vi "build.key.maps.vi"() -> ()   [LabVIEW 2024]
uses:
  definitions/comicvine_issue.generic_credit.ctl
  definitions/local_issue.ctl
  definitions/comicvine_issue.associated_image.ctl
  definitions/comicvine_issue.person_credit.ctl
  <vilib>/addons/_JKI.lib/Serialization/JSON/JKI JSON Serialization.lvlib
panel:
  out "progress":i32(slide) scale=0.0..21267.0
  out "current file":string
  in  "error in (no error)":errorcluster
  out "error out":errorcluster
  in  "storyArc map path":path=path "D:/Comics/data/key_maps/storyArc.json"
  in  "team map path":path=path "D:/Comics/data/key_maps/team.json"
  in  "character map path":path=path "D:/Comics/data/key_maps/char.json"
  in  "Folder Path":path=path "D:/Comics/data/cv_issues"
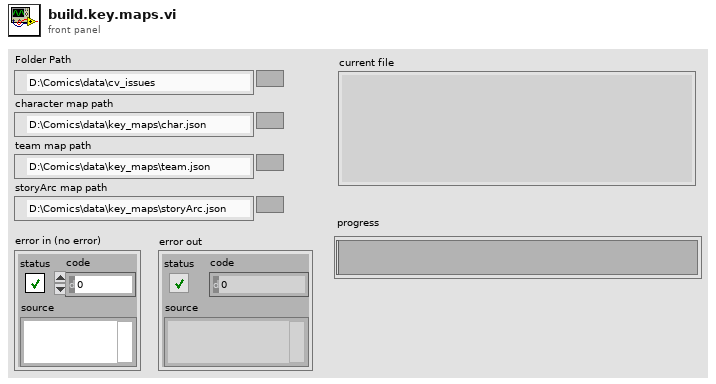
[diagram p1: front panel]
types:
  T1 = typedef "comicvine_issue.generic_credit.ctl" = cluster{"id":i32, "name":string}
  T2 = cluster{"map":cluster{"key":T1, "issue_ids":i32[]}[]}
  T3 = typedef "local_issue.ctl" = cluster{"cover_date":timestamp, "id":i32, "cv_id":string, "name":string, "sortable_name":string, "issue_number":string, "deck":string, "description":string, "volume":T1, "store_date":timestamp, "date_last_updated":timestamp, "site_detail_url":string, "cover_url":string, "associated_images":T4[], "characters":T1[], "concepts":T1[], "creators":T5[], "storyArcs":T1[], "teams":T1[]}
  T4 = typedef "comicvine_issue.associated_image.ctl" = cluster{"original_url":string, "id":i32}
  T5 = typedef "comicvine_issue.person_credit.ctl" = cluster{"id":i32, "name":string, "role":string}
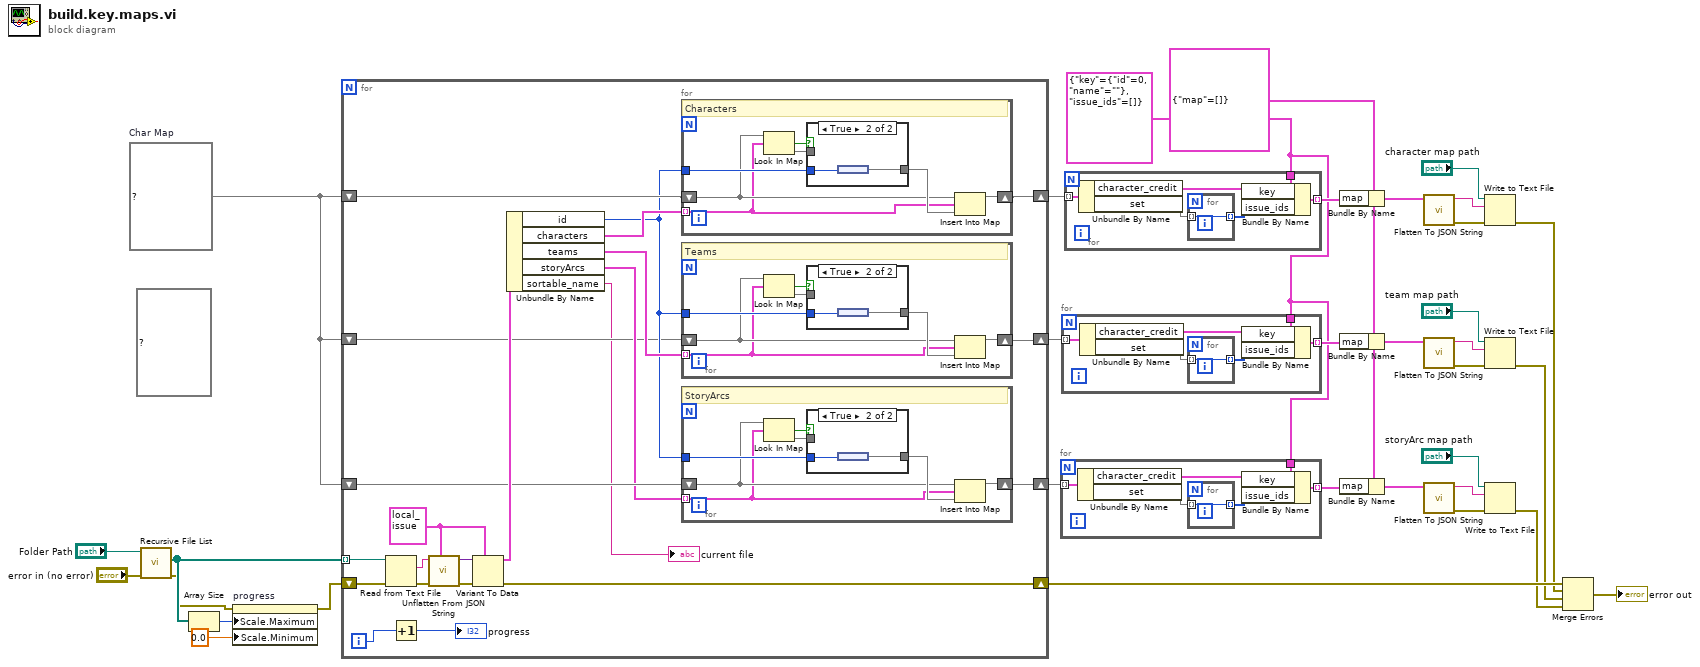
[diagram p0: block diagram]
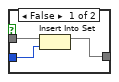
[diagram p2: hidden frame]
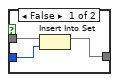
[diagram p3: hidden frame]
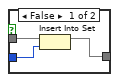
[diagram p4: hidden frame]
diagram:
  w6 = T2 {"map"=[]}
  w7 = cluster{"key":T1, "issue_ids":i32[]} {"key"={"id"=0, "name"=""}, "issue_ids"=[]}
  w8 = map{T1, set{i32}} {}  # Char Map
  (unwired) map{i32, set{i32}} {} ("map")
  n1 = call <vilib>:"Recursive File List.vi"("error in (no error)"="error in (no error)", "Folder Path"="Folder Path") -> ("error out"=w2:errorcluster, "All Files in Dir"=w5:path[])  [unwired: 5 in, 3 out]
  n2 = Array Size(array=w5) -> (size(s)=w4:i32)
  n3 = property on="progress" class="Slide (strict)"(error in=w2, "Scale.Maximum"=w4, "Scale.Minimum"=0.0 ("Scale.Range:Minimum")) -> (error out=w1:errorcluster)  [unwired: 1 in, 1 out]
  n4 = for {
    shift-right: [w48] -> w14
    shift-left: w1 -> [w54]
    tunnel: w5 -> [w55] mode=indexing
    shift-right: [w45] -> w32
    shift-left: w8 -> [w46]
    shift-right: [w39] -> w16
    shift-left: w8 -> [w37]
    shift-right: [w38] -> w15
    shift-left: w8 -> [w43]
    i -> [w35]
    w50 = T3 {"cover_date"=timestamp(0 s since 1904-01-01), "id"=0, "cv_id"="", "name"="", "sortable_name"="", "issue_number"="", "deck"="", "description"="", "volume"={"id"=0, "name"=""}, "store_date"=timestamp(0 s since 1904-01-01), "date_last_updated"=timestamp(0 s since 1904-01-01), "site_detail_url"="", "cover_url"="", "associated_images"=[], "characters"=[], "concepts"=[], "creators"=[], "storyArcs"=[], "teams"=[]} ("issue")
    n5 = Read from Text File(file (use dialog)=w55, error in=w54) -> (text=w52:string, error out=w53:errorcluster)  [unwired: 2 in, 2 out]
    n6 = Increment(x=w35) -> (x+1=→"progress":i32)
    n7 = call <vilib>:"Unflatten From JSON String.vi"("Type and Defaults"=w50, "error in"=w53, "JSON String"=w52) -> ("error out"=w49:errorcluster, "Variant"=w51:variant)  [unwired: 7 in]
    n8 = Variant To Data(error in=w49, type=w50, Variant=w51) -> (data=w47:T3, error out=w48:errorcluster)
    n9 = Unbundle By Name(w47) -> ("id"=w40:i32, "characters"=w44:T1[], "teams"=w41:T1[], "storyArcs"=w42:T1[], "sortable_name"=→"current file":string)
    n10 = for {
      tunnel: w44 -> [w80] mode=indexing
      shift-right: [w82] -> w45
      shift-left: w46 -> [w81]
      tunnel: w40 -> [w84]
      # "Characters"
      n11 = Look In Map(map=w81, key=w80) -> (key not found?=w86:bool, value=w85:set{i32})  [unwired: 1 in]
      n12 = case shown="True" w86 {
        tunnel: w85 -> [w89 _]
        tunnel: w84 -> [w88 w91]
        tunnel: [w87 w90] -> w83
        frame False {
          n13 = Insert Into Set(10:w88, 11:w89) -> (3:w87:set{i32})  [unwired: 1 out]
        }
        frame True {
          n14 = node(w91) -> (w90:set{i32})
        }
      }
      n15 = Insert Into Map(map in=w81, key=w80, value=w83) -> (map out=w82:map{T1, set{i32}})  [unwired: 2 out]
    }
    n16 = for {
      tunnel: w41 -> [w68] mode=indexing
      shift-right: [w70] -> w39
      shift-left: w37 -> [w69]
      tunnel: w40 -> [w72]
      # "Teams"
      n17 = Look In Map(map=w69, key=w68) -> (key not found?=w74:bool, value=w73:set{i32})  [unwired: 1 in]
      n18 = case shown="True" w74 {
        tunnel: w73 -> [w77 _]
        tunnel: w72 -> [w76 w79]
        tunnel: [w75 w78] -> w71
        frame False {
          n19 = Insert Into Set(10:w76, 11:w77) -> (3:w75:set{i32})  [unwired: 1 out]
        }
        frame True {
          n20 = node(w79) -> (w78:set{i32})
        }
      }
      n21 = Insert Into Map(map in=w69, key=w68, value=w71) -> (map out=w70:map{T1, set{i32}})  [unwired: 2 out]
    }
    n22 = for {
      tunnel: w42 -> [w56] mode=indexing
      shift-right: [w58] -> w38
      shift-left: w43 -> [w57]
      tunnel: w40 -> [w60]
      # "StoryArcs"
      n23 = Look In Map(map=w57, key=w56) -> (key not found?=w62:bool, value=w61:set{i32})  [unwired: 1 in]
      n24 = case shown="True" w62 {
        tunnel: w61 -> [w65 _]
        tunnel: w60 -> [w64 w67]
        tunnel: [w63 w66] -> w59
        frame False {
          n25 = Insert Into Set(10:w64, 11:w65) -> (3:w63:set{i32})  [unwired: 1 out]
        }
        frame True {
          n26 = node(w67) -> (w66:set{i32})
        }
      }
      n27 = Insert Into Map(map in=w57, key=w56, value=w59) -> (map out=w58:map{T1, set{i32}})  [unwired: 2 out]
    }
  }
  n28 = for {
    tunnel: w15 -> [w97] mode=indexing
    tunnel: w7 -> [w95]
    tunnel: [w92] -> w21 mode=indexing
    n29 = Unbundle By Name(w97) -> ("character_credit"=w94:T1, "set"=w96:set{i32})
    n30 = for {
      tunnel: w96 -> [w98] mode=indexing
      tunnel: [w98] -> w93 mode=indexing
    }
    n31 = Bundle By Name(cluster=w95, "key"=w94, "issue_ids"=w93) -> (w92:cluster{"key":T1, "issue_ids":i32[]})
  }
  n32 = for {
    tunnel: w16 -> [w104] mode=indexing
    tunnel: w7 -> [w102]
    tunnel: [w99] -> w22 mode=indexing
    n33 = Unbundle By Name(w104) -> ("character_credit"=w101:T1, "set"=w103:set{i32})
    n34 = for {
      tunnel: w103 -> [w105] mode=indexing
      tunnel: [w105] -> w100 mode=indexing
    }
    n35 = Bundle By Name(cluster=w102, "key"=w101, "issue_ids"=w100) -> (w99:cluster{"key":T1, "issue_ids":i32[]})
  }
  n36 = for {
    tunnel: w32 -> [w111] mode=indexing
    tunnel: w7 -> [w109]
    tunnel: [w106] -> w31 mode=indexing
    n37 = Unbundle By Name(w111) -> ("character_credit"=w108:T1, "set"=w110:set{i32})
    n38 = for {
      tunnel: w110 -> [w112] mode=indexing
      tunnel: [w112] -> w107 mode=indexing
    }
    n39 = Bundle By Name(cluster=w109, "key"=w108, "issue_ids"=w107) -> (w106:cluster{"key":T1, "issue_ids":i32[]})
  }
  n40 = Bundle By Name(cluster=w6, "map"=w31) -> (w30:T2)
  n41 = Bundle By Name(cluster=w6, "map"=w22) -> (w23:T2)
  n42 = Bundle By Name(cluster=w6, "map"=w21) -> (w20:T2)
  n43 = call <vilib>:"Flatten To JSON String.vi"("Variant"=w30) -> ("error out"=w29:errorcluster, "JSON String"=w28:string)  [unwired: 9 in]
  n44 = call <vilib>:"Flatten To JSON String.vi"("Variant"=w23) -> ("error out"=w24:errorcluster, "JSON String"=w25:string)  [unwired: 9 in]
  n45 = call <vilib>:"Flatten To JSON String.vi"("Variant"=w20) -> ("error out"=w19:errorcluster, "JSON String"=w18:string)  [unwired: 9 in]
  n46 = Write to Text File(file (use dialog)="character map path", text=w28, error in=w29) -> (error out=w13:errorcluster)  [unwired: 1 in, 2 out]
  n47 = Write to Text File(file (use dialog)="team map path", text=w25, error in=w24) -> (error out=w12:errorcluster)  [unwired: 1 in, 2 out]
  n48 = Write to Text File(file (use dialog)="storyArc map path", text=w18, error in=w19) -> (error out=w11:errorcluster)  [unwired: 1 in, 2 out]
  n49 = Merge Errors(w14, w13, w12, w11) -> (→"error out":errorcluster)
